vi "Periodic Tasks.vi"(8 "error in":errorcluster) -> ()   [LabVIEW 2015]
doc: "This VI runs in parallel to other tasks. It can contain as many user-defined periodic loops as you need. These can carry out PID or other sorts of timed response."
uses:
  <vilib>/Rock Robotics/WPI/Solenoid/WPI_SolenoidChannel.ctl
  <vilib>/Rock Robotics/SystemInterfaces/DIO/FPGA_DIOChannel.ctl
  <vilib>/Rock Robotics/SystemInterfaces/AI/FPGA_AIChannel.ctl
  <vilib>/Rock Robotics/SystemInterfaces/i2clib/i2c_bus.ctl
  <vilib>/Rock Robotics/WPI/Solenoid/WPI_SolenoidValue.ctl
  <vilib>/Rock Robotics/WPI/Utilities/WPI_GetSetVariantRefNum.vi
  <vilib>/Rock Robotics/Network Tables/SD Read Number.vi
  <vilib>/Rock Robotics/Network Tables/SD Write Number.vi
  <vilib>/Rock Robotics/WPI/Solenoid/WPI_SolenoidOpenDouble.vi
  Robot Global Data.vi
  <vilib>/Rock Robotics/WPI/Solenoid/WPI_SolenoidSetEnum.vi
panel:
  in  "Limit Switch Channel":T1=enum."DIO 9"
  in  "Retract Solenoid Channel":T2
  in  "Extend Solenoid Channel":T2=enum."Solenoid 1"
  in  "stop":bool
  out "Compressor Monitoring":bool
  in  "Auto Retract":bool
  out "Cylinder Limit":bool
  out "Compressor Running":bool
  in  "Red":u32(colorbox)
  in  "Green":u32(colorbox)
  in  "Yellow":u32(colorbox)
  out "Waveform Chart 3":u8(graph)
  out "Waveform Chart 2":u8(graph)
  out "Waveform Chart":u8(graph)
  in  "I2CBytesToRead":u8
  out "Data Out":u8[](array[numeric])
  out "LED_OFF":u32(colorbox)=16775840
  out "LED_ON":u32(colorbox)=65282
  in  "error in (no error)":errorcluster
  out "error out":errorcluster
  in  "Brightness":u8(slide)=255 scale=0.0..255.0
  out "LED Position":u8(slide)=7 scale=0.0..30.0
  in  "Position Speed":u32(slide)=20 scale=5.0..2000.0
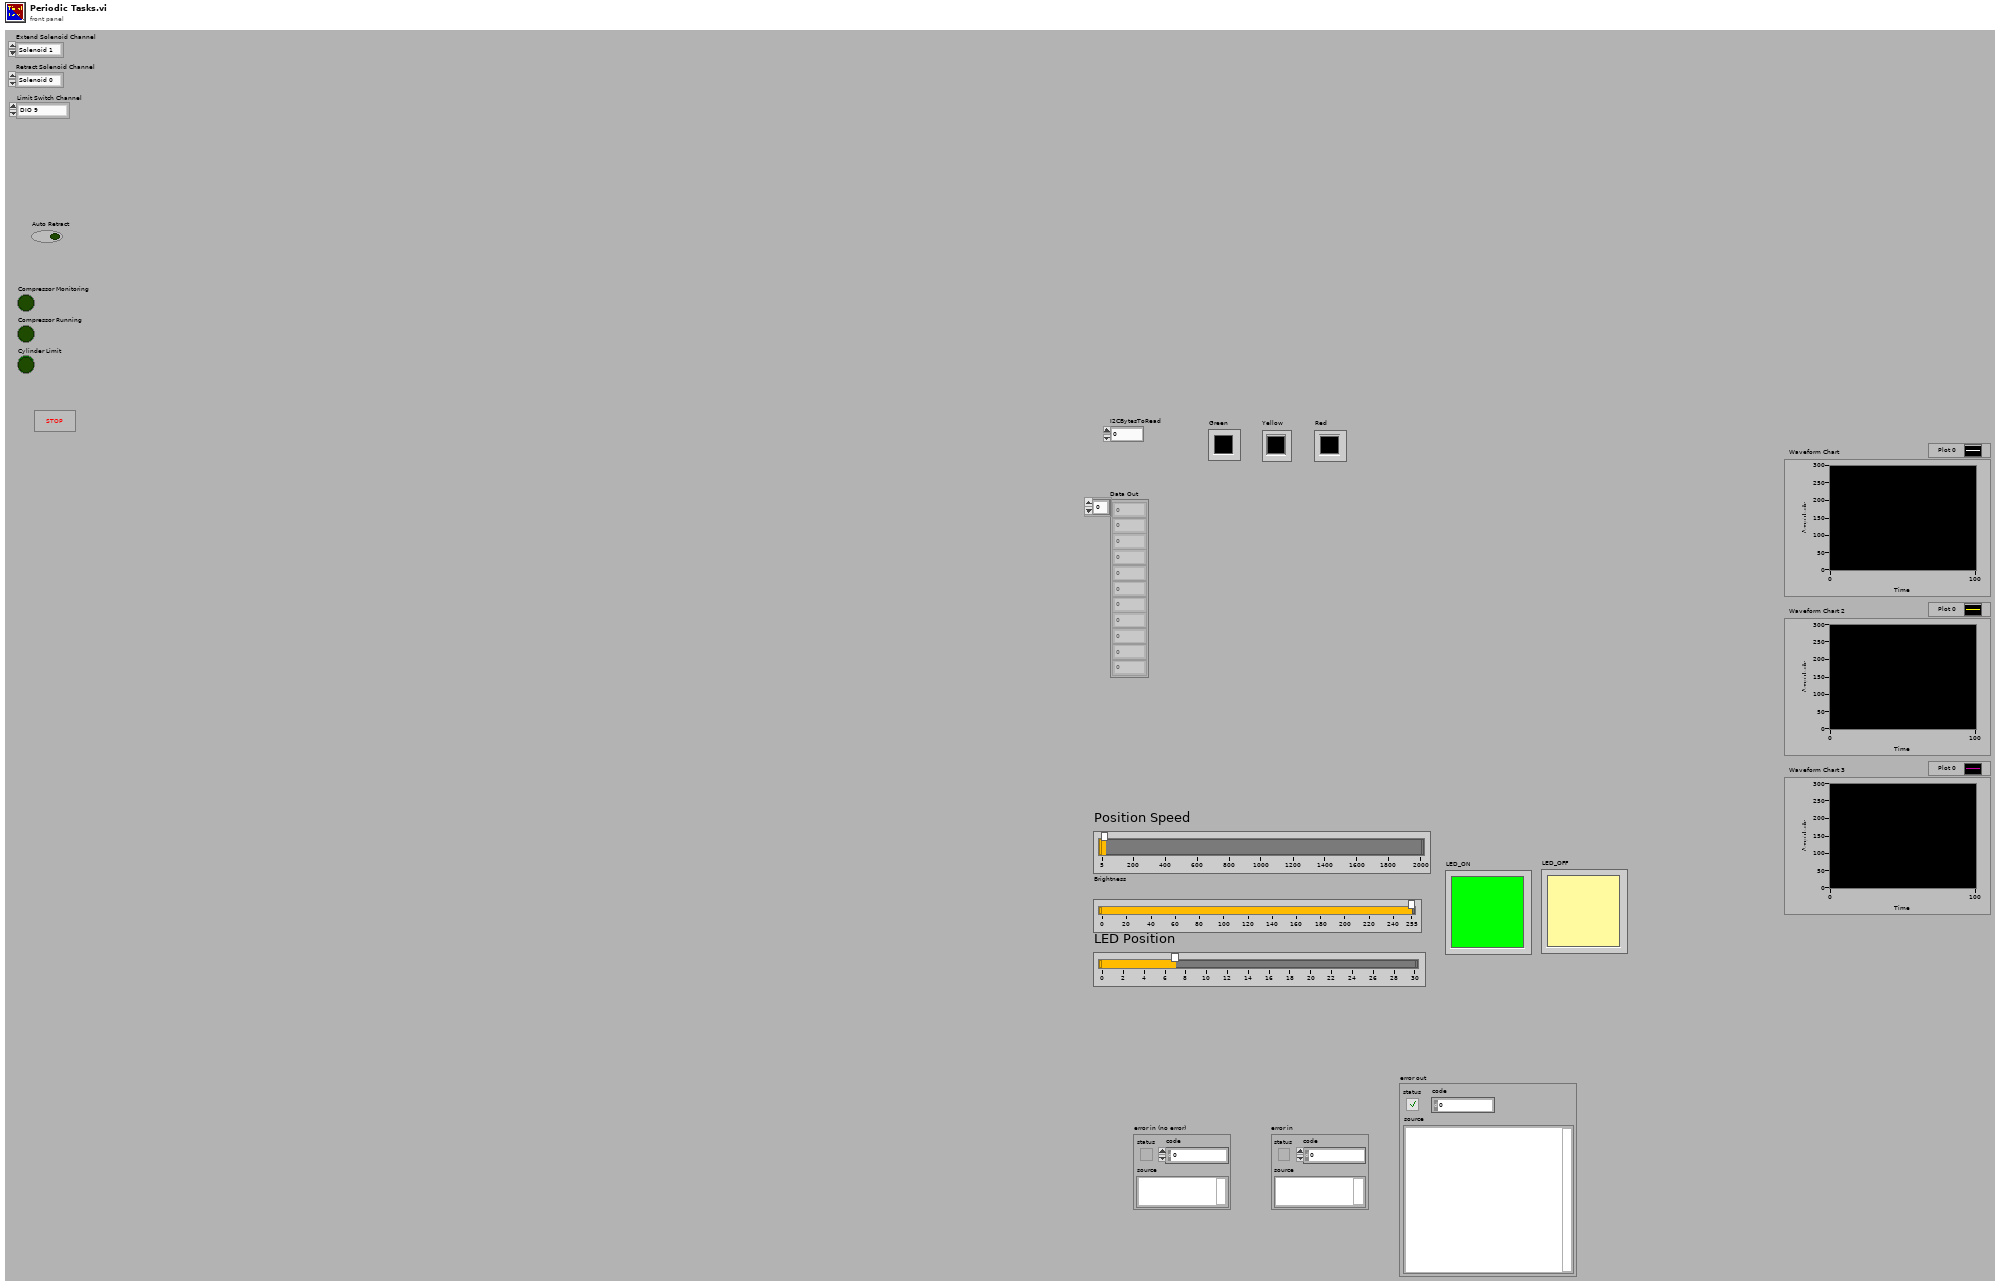
[diagram p1: front panel]
types:
  T1 = typedef "FPGA_DIOChannel.ctl" = enum8{"DIO 0", "DIO 1", "DIO 2", "DIO 3", "DIO 4", "DIO 5", "DIO 6", "DIO 7", "DIO 8", "DIO 9", "DIO MXP 0", "DIO MXP 1", "DIO MXP 2", "DIO MXP 3", "DIO MXP 4", "DIO MXP 5", "DIO MXP 6", "DIO MXP 7", "DIO MXP 8", "DIO MXP 9", "DIO MXP 10", "DIO MXP 11", "DIO MXP 12", "DIO MXP 13", "DIO MXP 14", "DIO MXP 15", "Invalid"}
  T2 = typedef "WPI_SolenoidChannel.ctl" = enum8{"Solenoid 0", "Solenoid 1", "Solenoid 2", "Solenoid 3", "Solenoid 4", "Solenoid 5", "Solenoid 6", "Solenoid 7", "Invalid"}
  T3 = typedef "i2c_bus.ctl" = enum16{"I2C On-Board", "I2C MXP", "Invalid"}
  T4 = typedef "FPGA_AIChannel.ctl" = enum8{"AI 0", "AI 1", "AI 2", "AI 3", "AI MXP 0", "AI MXP 1", "AI MXP 2", "AI MXP 3", "Invalid"}
  T5 = typedef "WPI_I2CDevRef.ctl" = cluster{"DevStatus":errorcluster, "Device Address":u8, "Handle":i32, "I2C Bus":T3}
  T6 = typedef "WPI_AnalogChannelDevRef.ctl" = cluster{"DevStatus":errorcluster, "Analog Channel":T4}
  T7 = typedef "WPI_JoystickDevRef.ctl" = cluster{"Device":T8}
  T8 = typedef "WPI_JoystickDeviceEnum.ctl" = enum16{"USB 0", "USB 1", "USB 2", "USB 3", "USB 4", "USB 5"}
  T9 = typedef "WPI_RobotDriveDevRef.ctl" = cluster{"DevStatus":errorcluster, "Motors[]":T10[], "Square Inputs":bool, "Max Output":dbl}
  T10 = typedef "WPI_MotorControlDeviceRef.ctl" = cluster{"DeviceStatus":errorcluster, "Type":T11, "PWM":cluster{"PWM Channel":T12, "DeadBand":T13}, "CAN":cluster{"Device Number":u8, "Control Mode":T14, "Semaphore":T15, "Max Vout":dbl, "TalonSRX Control Mode":T16}, "Invert":bool}
  T11 = typedef "WPI_MotorControlType.ctl" = enum16{"PWM", "CAN", "CANTalonSRX"}
  T12 = typedef "FPGA_DIOPWMChannel.ctl" = enum8{"PWM 0", "PWM 1", "PWM 2", "PWM 3", "PWM 4", "PWM 5", "PWM 6", "PWM 7", "PWM 8", "PWM 9", "PWM MXP 0", "PWM MXP 1", "PWM MXP 2", "PWM MXP 3", "PWM MXP 4", "PWM MXP 5", "PWM MXP 6", "PWM MXP 7", "PWM MXP 8", "PWM MXP 9", "Invalid"}
  T13 = typedef "WPI_PWMDeadband.ctl" = cluster{"Name":string, "maxPositivePwm":i32, "minPositivePwm":i32, "centerPwm":i32, "maxNegativePwm":i32, "minNegativePwm":i32, "angularRange":u16}
  T14 = typedef "WPI_CANJaguar_ControlMode.ctl" = enum8{"Percent VBus", "Current", "Speed", "Position", "Voltage"}
  T15 = typedef "Semaphore RefNum" = refnum<k1>
  T16 = typedef "WPI_CANTalonSRX_APIControlMode.ctl" = enum8{"Percent VBus", "Speed", "Position", "Slave", "Unchanged / Invalid", "Voltage Compensation", "Current", "Motion Profile"}
  T17 = cluster{"JoystickDevRef":T7, "RobotDriveDevRef":T9}
  T18 = typedef "WPI_CompressorDevRef.ctl" = cluster{"DevStatus":errorcluster, "Pneumatics Control Module":u8}
  T19 = typedef "WPI_DigitalInputDevRef.ctl" = cluster{"DevStatus":errorcluster, "DIO Channel":T1}
  T20 = typedef "WPI_SolenoidDevRef.ctl" = cluster{"DevStatus":errorcluster, "Pneumatics Control Module":u8, "Forward Solenoid Channel":T2, "Reverse Solenoid Channel":T2}
  T21 = typedef "WPI_SolenoidValue.ctl" = enum16{"Off", "On", "Forward", "Reverse"}
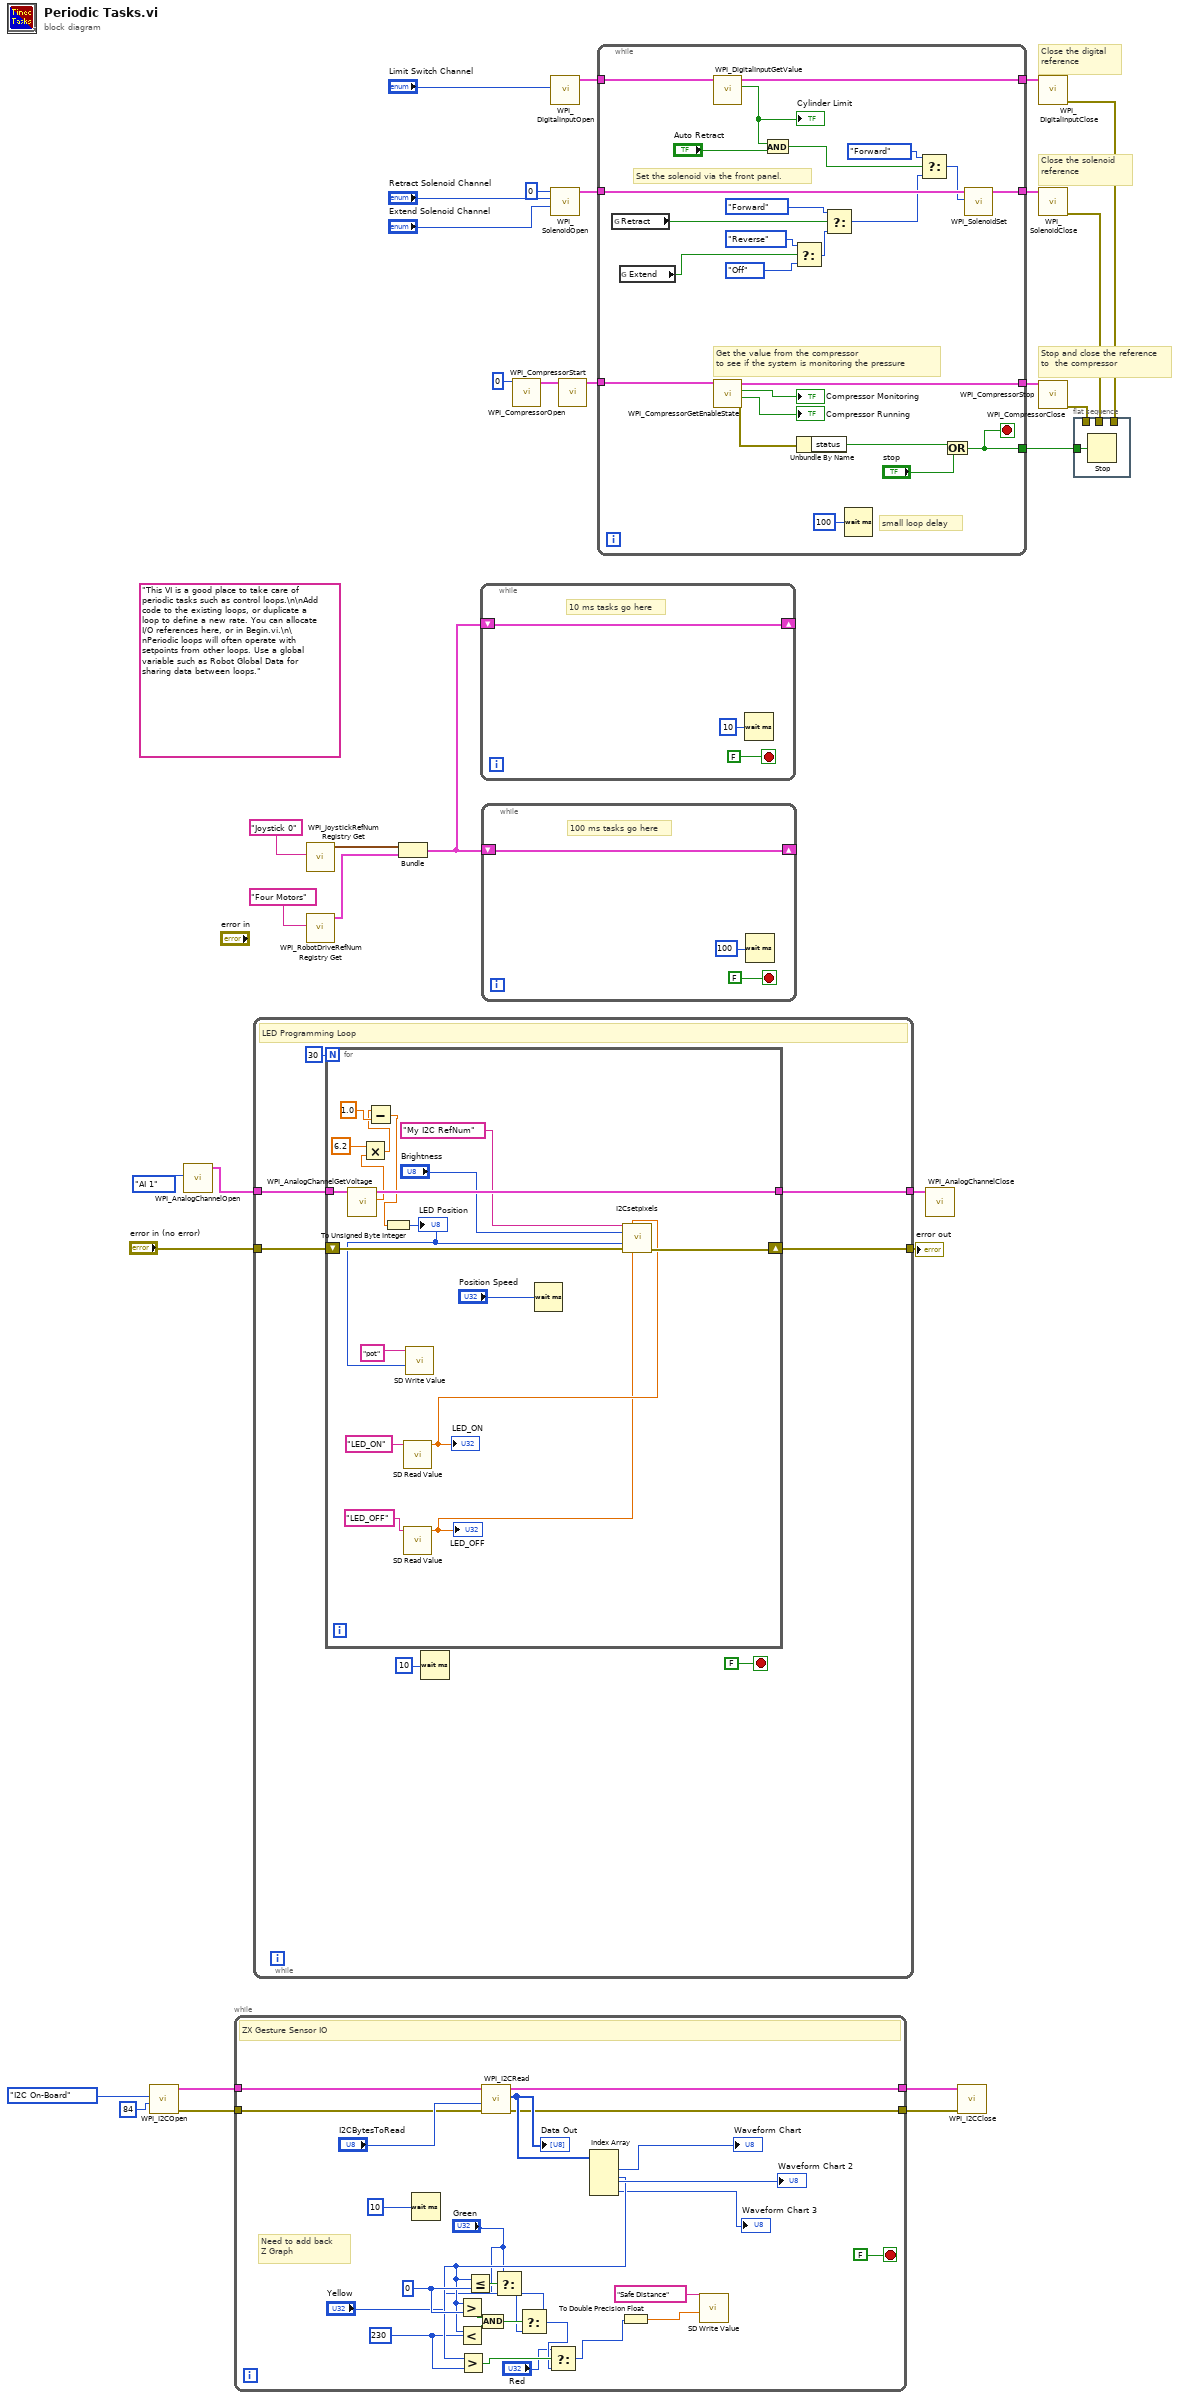
[diagram p0: block diagram]
diagram:
  (unwired) "This VI is a good place to take care of periodic tasks such as control loops.\n\nAdd code to the existing loops, or duplicate a loop to define a new rate. You can allocate I/O references here, or in Begin.vi.\n\nPeriodic loops will often operate with setpoints from other loops. Use a global variable such as Robot Global Data for sharing data between loops."
  # "Close the digital\nreference"
  # "Close the solenoid\nreference"
  # "Stop and close the reference to  the compressor"
  n1 = call <vilib>:"WPI_I2COpen.vi"("Device Address"=u8 84, "I2C Bus"=i2c_bus."I2C On-Board") -> ("error out"=w19:errorcluster, "I2CDevRef"=w21:T5)  [unwired: 8 in]
  n2 = call <vilib>:"WPI_AnalogChannelOpen.vi"("Analog Channel"=FPGA_AIChannel."AI 1") -> ("AIDeviceRef"=w25:T6)  [unwired: 9 in, 1 out]
  n3 = while {
    tunnel: w21 -> [w58]
    tunnel: [w57] -> w20
    tunnel: w19 -> [w54]
    tunnel: [w53] -> w18
    stop <- FALSE stop-if-true
    w49 = 0
    w45 = 230
    # "Need to add back \nZ Graph"
    # "ZX Gesture Sensor IO"
    n4 = Wait (ms)(milliseconds to wait=u32 10) -> ()  [unwired: 1 out]
    n5 = call <vilib>:"WPI_I2CRead.vi"("error in (no error)"=w54, "I2CBytesToRead"="I2CBytesToRead", "I2CDevRef"=w58) -> ("error out"=w53:errorcluster, "Data Out"=w60:u8[], "I2CDevRef"=w57:T5)  [unwired: 6 in]
    "Data Out" <- w60
    n6 = Index Array(array=w60) -> (element #1=→"Waveform Chart":u8, element #2=w46:u8, element #3=→"Waveform Chart 2":u8, element #4=→"Waveform Chart 3":u8)  [unwired: 4 in]
    n7 = Greater?(x=w46, y=w49) -> (0:w48:bool)
    n8 = Less?(x=w46, y=w45) -> (x < y?=w47:bool)
    n9 = Greater?(x=w46, y=w45) -> (0:w44:bool)
    n10 = Less Or Equal?(x=w46, y=w49) -> (x <= y?=w42:bool)
    n11 = And(x=w48, y=w47) -> (x .and. y?=w43:bool)
    n12 = Select(t="Green", s=w42, f="Green") -> (s? t:f=w41:u32)
    n13 = Select(t="Yellow", s=w43, f=w41) -> (s? t:f=w38:u32)
    n14 = Select(t="Red", s=w44, f=w38) -> (s? t:f=w36:u32)
    n15 = To Double Precision Float(number=w36) -> (double precision float=w35:dbl)
    n16 = call-poly <vilib>:"SD Write Value.vi"("Numeric"=w35, "Name"="Safe Distance") -> ()  [unwired: 8 in, 2 out]
  }
  n17 = while {
    tunnel: "error in (no error)" -> [w66]
    tunnel: [w63] -> w27
    tunnel: w25 -> [w62]
    tunnel: [w61] -> w24
    stop <- FALSE stop-if-true
    # "LED Programming Loop"
    n18 = for {
      N: 30 -> [_]
      shift-right: [w74] -> w63
      shift-left: w66 -> [w75]
      tunnel: w62 -> [w84]
      tunnel: [w83] -> w61
      n19 = call <vilib>:"WPI_AnalogChannelGetVoltage.vi"("AIDeviceRef"=w84) -> ("Voltage"=w81:dbl, "AIDeviceRef"=w83:T6)  [unwired: 8 in, 1 out]
      n20 = Multiply(x=6.2, y=w81) -> (x*y=w79:dbl)
      n21 = Subtract(x=w79, y=1.0 ("x")) -> (x-y=w78:dbl)
      n22 = To Unsigned Byte Integer(number=w78) -> (unsigned 8bit integer=w72:u8)
      "LED Position" <- w72
      n23 = call-poly <vilib>:"SD Read Value.vi"("Name"="LED_ON") -> ("Numeric"=w70:dbl)  [unwired: 8 in, 2 out]
      "LED_ON" <- w70
      n24 = call-poly <vilib>:"SD Read Value.vi"("Name"="LED_OFF") -> ("Numeric"=w68:dbl)  [unwired: 8 in, 2 out]
      "LED_OFF" <- w68
      n25 = call-poly <vilib>:"SD Write Value.vi"("Numeric"=w72, "Name"="pot") -> ()  [unwired: 8 in, 2 out]
      n26 = Wait (ms)(milliseconds to wait="Position Speed") -> ()  [unwired: 1 out]
      n27 = call "I2Csetpixels.vi"("I2C Reference In"="My I2C RefNum" ("refnum name"), "Color Box - On"=w70, "Brightness (0-255)"="Brightness", "LED Position"=w72, "Error In"=w75, "Color Box - Off"=w68) -> ("Error Out"=w74:errorcluster)  [unwired: 8 in, 1 out]
    }
    n28 = Wait (ms)(milliseconds to wait=u32 10) -> ()  [unwired: 1 out]
  }
  "error out" <- w27
  n29 = call <vilib>:"WPI_JoystickRefNum Registry Get.vi"("refnum name"="Joystick 0") -> ("JoystickDevRef"=w31:T7)  [unwired: 1 in, 9 out]
  n30 = call <vilib>:"WPI_RobotDriveRefNum Registry Get.vi"("refnum name"="Four Motors") -> ("RobotDriveDevRef"=w30:T9)  [unwired: 1 in, 9 out]
  n31 = Bundle("JoystickDevRef"=w31, "RobotDriveDevRef"=w30) -> (w29:T17)  [unwired: 1 out]
  n32 = while {
    shift-right: [w86] -> _
    shift-left: w29 -> [w86]
    stop <- FALSE stop-if-true
    # "10 ms tasks go here"
    n33 = Wait (ms)(milliseconds to wait=u32 10) -> ()  [unwired: 1 out]
  }
  n34 = while {
    shift-right: [w89] -> _
    shift-left: w29 -> [w89]
    stop <- FALSE stop-if-true
    # "100 ms tasks go here"
    n35 = Wait (ms)(milliseconds to wait=u32 100) -> ()  [unwired: 1 out]
  }
  n36 = call <vilib>:"WPI_CompressorOpen.vi"("Pneumatics Control Module (0)"=u8 0) -> ("CompressorDevRef"=w7:T18)  [unwired: 13 in, 1 out]
  n37 = call <vilib>:"WPI_DigitalInputOpen.vi"("DIO Channel"="Limit Switch Channel") -> ("DigitalInputDevRef"=w11:T19)  [unwired: 1 in, 9 out]
  n38 = call-poly <vilib>:"WPI_SolenoidOpen.vi"("Reverse Solenoid Channel"="Extend Solenoid Channel", "Forward Solenoid Channel"="Retract Solenoid Channel", "Pneumatics Control Module (0)"=u8 0) -> ("SolenoidDevRef"=w13:T20)  [unwired: 1 in, 7 out]
  n39 = call <vilib>:"WPI_CompressorStart.vi"("CompressorDevRef"=w7) -> ("CompressorDevRef"=w16:T18)  [unwired: 1 in, 9 out]
  n40 = while {
    tunnel: w16 -> [w116]
    tunnel: [w115] -> w15
    tunnel: [w113] -> w6
    tunnel: w13 -> [w108]
    tunnel: [w100] -> w14
    tunnel: w11 -> [w107]
    tunnel: [w106] -> w10
    stop <- w113 stop-if-true
    # "small loop delay"
    # "Get the value from the compressor \nto see if the system is monitoring the pressure"
    # "Set the solenoid via the front panel."
    n41 = global read "Robot Global Data.vi" "Retract"() -> (w92:bool)
    n42 = global read "Robot Global Data.vi" "Extend"() -> (w93:bool)
    n43 = call <vilib>:"WPI_DigitalInputGetValue.vi"("DigitalInputDevRef"=w107) -> ("Value"=w98:bool, "DigitalInputDevRef"=w106:T19)  [unwired: 1 in, 8 out]
    "Cylinder Limit" <- w98
    n44 = call <vilib>:"WPI_CompressorGetEnableState.vi"("CompressorDevRef"=w116) -> ("error out"=w111:errorcluster, "Compressor Running"=→"Compressor Running":bool, "Enabled"=→"Compressor Monitoring":bool, "CompressorDevRef"=w115:T18)  [unwired: 1 in, 6 out]
    n45 = And(x=w98, y="Auto Retract") -> (x .and. y?=w94:bool)
    n46 = Select(t=WPI_SolenoidValue."Reverse" ("Value"), s=w93, f=WPI_SolenoidValue."Off" ("Value")) -> (s? t:f=w102:T21)
    n47 = Unbundle By Name(w111) -> ("status"=w110:bool)
    n48 = Select(t=WPI_SolenoidValue."Forward" ("Value"), s=w92, f=w102) -> (s? t:f=w95:T21)
    n49 = Wait (ms)(milliseconds to wait=u32 100) -> ()  [unwired: 1 out]
    n50 = Select(t=WPI_SolenoidValue."Forward" ("Value"), s=w94, f=w95) -> (s? t:f=w96:T21)
    n51 = Or(x=w110, y="stop") -> (x .or. y?=w113:bool)
    n52 = call-poly <vilib>:"WPI_SolenoidSet.vi"("Value"=w96, "SolenoidDevRef"=w108) -> ("SolenoidDevRef"=w100:T20)  [unwired: 1 in, 8 out]
  }
  n53 = call <vilib>:"WPI_AnalogChannelClose.vi"("AIDeviceRef"=w24) -> ()  [unwired: 10 in, 1 out]
  n54 = call <vilib>:"WPI_I2CClose.vi"("error in (no error)"=w18, "I2CDevRef"=w20) -> ()  [unwired: 9 in, 1 out]
  n55 = call <vilib>:"WPI_DigitalInputClose.vi"("DigitalInputDevRef"=w10) -> ("error out"=w3:errorcluster)  [unwired: 1 in, 9 out]
  n56 = call <vilib>:"WPI_SolenoidClose.vi"("SolenoidDevRef"=w14) -> ("error out"=w4:errorcluster)  [unwired: 1 in, 9 out]
  n57 = call <vilib>:"WPI_CompressorStop.vi"("CompressorDevRef"=w15) -> ("CompressorDevRef"=w17:T18)  [unwired: 1 in, 9 out]
  n58 = call <vilib>:"WPI_CompressorClose.vi"("CompressorDevRef"=w17) -> ("error out"=w5:errorcluster)  [unwired: 1 in, 9 out]
  n59 = flat-sequence {
    tunnel: w6 -> [w117]
    tunnel: w5 -> [_]
    tunnel: w4 -> [_]
    tunnel: w3 -> [_]
    frame #0 {
      n60 = Stop(stop? (T)=w117) -> ()
    }
  }
